vi "PIMAX_2.vi"() -> ()   [LabVIEW 2018]
uses:
  <vilib>/Enthought/Python Integration Toolkit/api/Console Visibility.ctl
  Global Variables.vi
  <vilib>/Enthought/Python Integration Toolkit/Python Integration Toolkit.lvlib
panel:
  in  "Settings":T1(array[cluster])=[{"Camera Setup"=enum."Imaging", "Acuisition type"=enum."Repetitive", "Gate Width"=10000.0, "Gate Start"=200.0, "# Frames"=1, "Center \nWavelength"=790.0, "# Acquisitions"=100, "Exposures per frame"=10}, {"Camera Setup"=enum."Imaging", "Acuisition type"=enum."Sequential", "Gate Width"=300.0, "Gate Start"=200.0, "# Frames"=20, "Center \nWavelength"=790.0, "# Acquisitions"=10, "Exposures per frame"=10}] {"# Acquisitions" min=1; "# Frames" min=1; "Gate Start" min=1.0 format="%#_13g"; "Gate Width" min=0.5 format="%#_13g"}
  out "Index Values":u32[](array[numeric])
  in  "Experiment Name":string="Imaging"
  in  "Logfile?":bool
  in  "File Path":path=path "F:/Data/Raw Data/2018-11-14/UnspecifiedProj/Temp Dependence/PIMAX_2_400C_3"
  in  "stop":bool
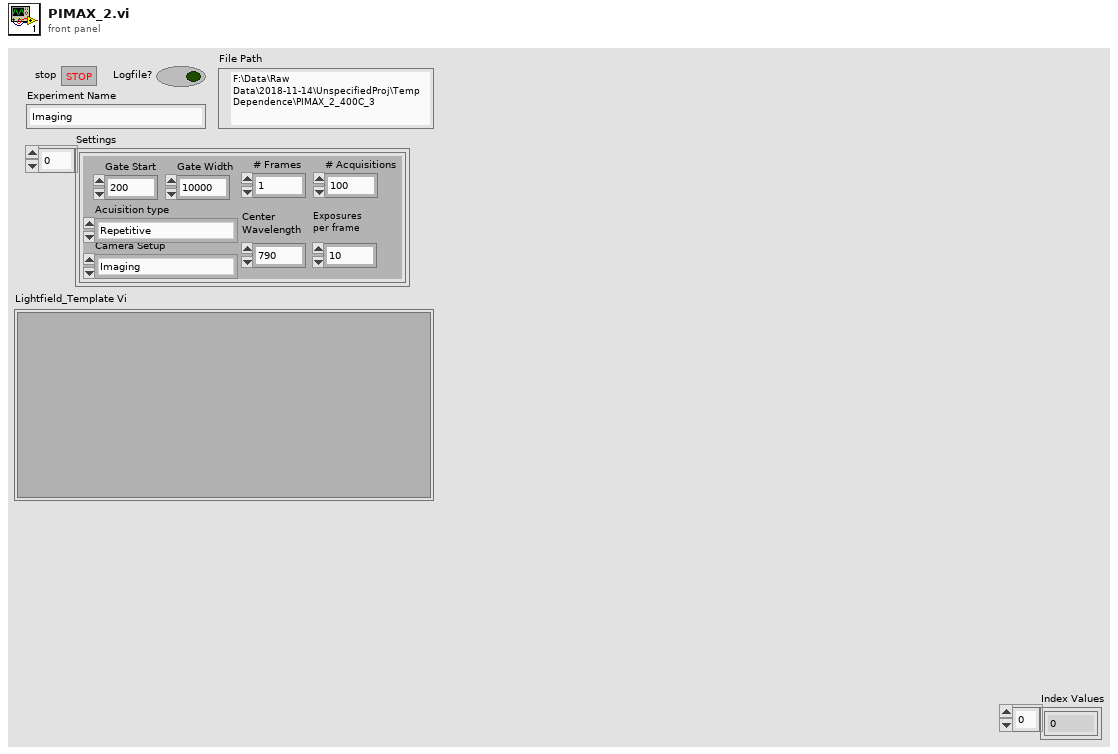
[diagram p1: front panel]
types:
  T1 = cluster{"Camera Setup":enum16{"Imaging", "Spectral"}, "Acuisition type":enum16{"Repetitive", "Sequential"}, "Gate Width":dbl, "Gate Start":dbl, "# Frames":i32, "Center \nWavelength":dbl, "# Acquisitions":i32, "Exposures per frame":i32}[]
  T2 = typedef "Python Integration Toolkit.lvlib/Console Visibility.ctl" = enum16{"Show Console", "Show Console While Running", "Hide Console"}
  T3 = enum32{"Bad", "Idle", "Run top level", "Running"}
  T4 = typedef "Python Integration Toolkit.lvlib/Session ID.ctl" = u64
  T5 = cluster{"Project":u16, "SubFolder":string, "Filename (Meas. Description)":string, "Measurement index":i32}
  T6 = typedef "Python Integration Toolkit.lvlib/Python Objects.ctl" = variant
  T7 = cluster{"Camera Setup":enum16{"Imaging", "Spectral"}, "Acuisition type":enum16{"Repetitive", "Sequential"}, "Gate Width":dbl, "Gate Start":dbl, "# Frames":i32, "Center \nWavelength":dbl, "# Acquisitions":i32, "Exposures per frame":i32}
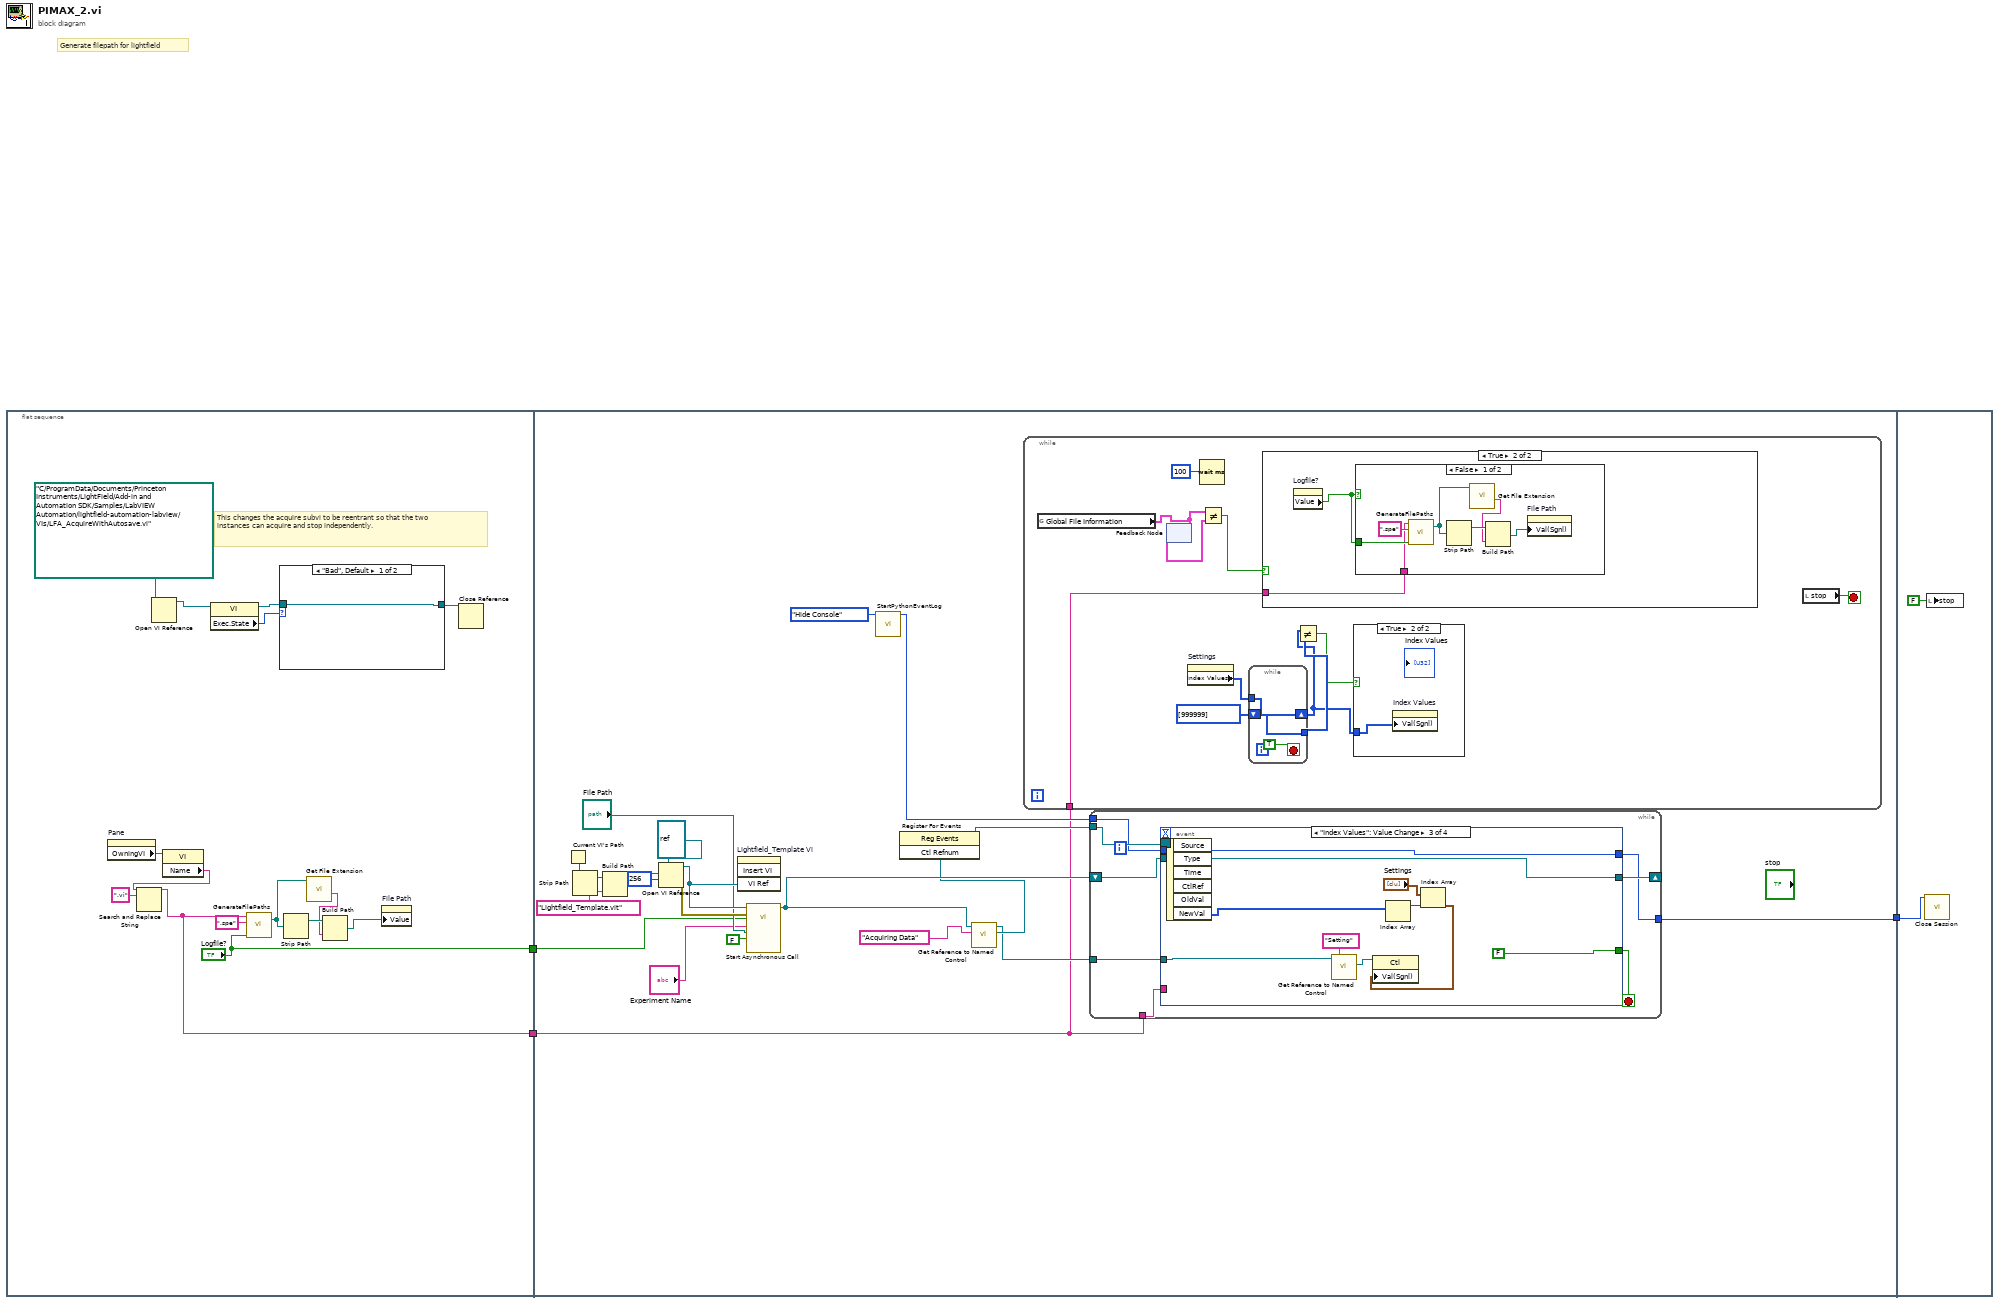
[diagram p0: block diagram]
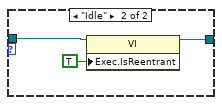
[diagram p2: hidden frame]
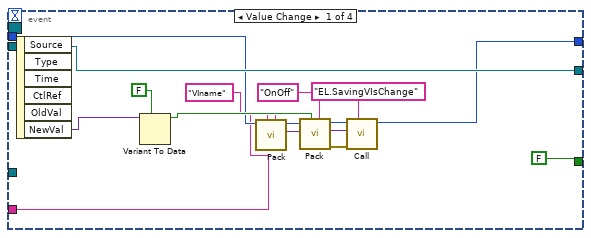
[diagram p6: hidden frame]
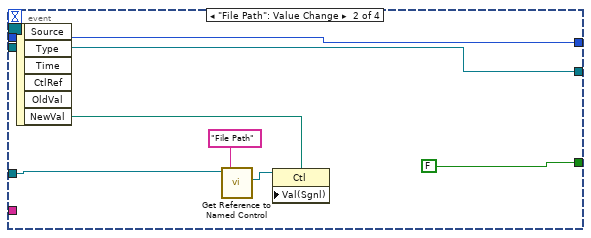
[diagram p7: hidden frame]
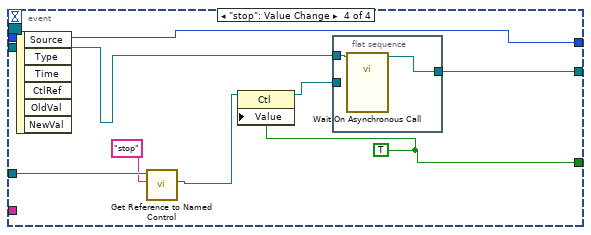
[diagram p8: hidden frame]
diagram:
  # "Generate filepath for lightfield"
  n1 = flat-sequence {
    tunnel: [w5] -> w2
    tunnel: ["Logfile?"] -> w1
    tunnel: [w32] -> w3
    tunnel: w2 -> [w25]
    tunnel: w1 -> [w24]
    tunnel: w3 -> [w119]
    frame #0 {
      # "This changes the acquire subvi to be reentrant so that the two instances can acquire and stop independently."
      n2 = property on="Pane" class="Pane"() -> ("OwningVI"=w8:refnum<vi>)  [unwired: 2 in, 2 out]
      n3 = Open VI Reference(vi path=path "C:/ProgramData/Documents/Princeton Instruments/LightField/Add-in and Automation SDK/Samples/LabVIEW Automation/lightfield-automation-labview/VIs/LFA_AcquireWithAutosave.vi") -> (vi reference=w11:refnum<vi>)  [unwired: 5 in, 1 out]
      n4 = property class="VI"(reference=w8) -> ("Name"=w6:string)  [unwired: 1 in, 2 out]
      n5 = Search and Replace String(input string=w6, search string=".vi") -> (result string=w5:string)  [unwired: 6 in, 3 out]
      n6 = property class="VI"(reference=w11) -> (reference out=w9:refnum<vi>, "Exec.State"=w10:T3)  [unwired: 1 in, 1 out]
      n7 = call "GenerateFilePaths.vi"("Logfile? (F)"="Logfile?", "Extension (.tdms)"=".spe" ("Extension"), "Device Name"=w5) -> ("Path"=w15:path)  [unwired: 2 in]
      n8 = case shown="\"Bad\", Default" w10 {
        tunnel: [w19 w21] -> w17
        tunnel: w9 -> [w19 w20]
        frame "Bad", Default {
        }
        frame "Idle" {
          n9 = property class="VI"(reference=w20, "Exec.IsReentrant"=TRUE ("Execution:Is Reentrant")) -> (reference out=w21:refnum<vi>)  [unwired: 1 in, 1 out]
        }
      }
      n10 = Strip Path(path=w15) -> (stripped path=w14:path)  [unwired: 1 out]
      n11 = call <vilib>:"Get File Extension.vi"("file"=w15) -> ("filename without extension"=w13:string)  [unwired: 6 in, 4 out]
      n12 = Build Path(base path=w14, name or relative path=w13) -> (appended path=w12:path)
      n13 = property on="File Path" class="Path"("Value"=w12) -> ()  [unwired: 2 in, 2 out]
      n14 = Close Reference(reference=w17) -> ()  [unwired: 1 in, 1 out]
    }
    frame #1 {
      n15 = Current VI's Path() -> (path=w42:path)
      n16 = Strip Path(path=w42) -> (stripped path=w43:path)  [unwired: 1 out]
      n17 = Build Path(base path=w43, name or relative path="Lightfield_Template.vit") -> (appended path=w39:path)
      n18 = Open VI Reference(type specifier VI Refnum (for type only)=refnum<vi> refnum, vi path=w39, options=256) -> (vi reference=w38:refnum<vi>, error out=w37:errorcluster)  [unwired: 1 in, 2 out]
      n19 = invoke on="Lightfield_Template Vi" class="SubPnl" method="Insert VI"("VI Ref"=w38) -> ()  [unwired: 3 in, 4 out]
      n20 = call-by-ref "Start Asynchronous Call"(reference=w38, error in=w37, "Add Time to filename"=w24, "Single Run"=FALSE, "File Path"="File Path", "Experiment Name"="Experiment Name") -> (reference out=w31:refnum<vi>)  [unwired: 8 in, 1 out]
      n21 = call "StartPythonEventLog.vi"("Console Visibility"=Console_Visibility."Hide Console") -> ("Session ID out"=w33:T4)  [unwired: 10 in]
      n22 = call "Get Reference to Named Control.vi"("Control Name"="Acquiring Data" ("element"), "Front Panel Ref"=w31) -> ("Ctl Refnum"=w29:refnum<vi>, "Panel Ref Out"=w28:refnum<vi>)  [unwired: 7 in, 1 out]
      n23 = register-events(w29) -> (reference out=w34:refnum<event-registration>)  [unwired: 2 in, 1 out]
      n24 = while {
        tunnel: w25 -> [w49]
        stop <- w54 stop-if-true
        n25 = global read "Global Variables.vi" "Global File Information"() -> (w52:T5)
        n26 = feedback #1() -> (w51:T5)  [unwired: 1 in]
        n27 = feedback-in #1(w52) -> ()
        n28 = property on="Settings" class="Arr (strict)"() -> ("Index Values"=w47:u32[])  [unwired: 2 in, 2 out]
        n29 = Wait (ms)(milliseconds to wait=100) -> ()  [unwired: 1 out]
        n30 = Not Equal?(x=w52, y=w51) -> (x != y?=w50:bool)
        n31 = while {
          tunnel: w47 -> [w58]
          shift-right: [w58] -> w44
          shift-left: u32[] [999999] ("Index Values") -> [w57]
          tunnel: [w57] -> w48
          stop <- TRUE stop-if-true
        }
        n32 = case shown="True" w50 {
          tunnel: w49 -> [_ w59]
          frame False {
          }
          frame True {
            n33 = property on="Logfile?" class="Bool (strict)"() -> ("Value"=w60:bool)  [unwired: 2 in, 2 out]
            n34 = case shown="False" w60 {
              tunnel: w60 -> [w63 _]
              tunnel: w59 -> [w61 _]
              frame False {
                n35 = call "GenerateFilePaths.vi"("Logfile? (F)"=w63, "Extension (.tdms)"=".spe" ("Extension"), "Device Name"=w61) -> ("Path"=w66:path)  [unwired: 2 in]
                n36 = Strip Path(path=w66) -> (stripped path=w65:path)  [unwired: 1 out]
                n37 = call <vilib>:"Get File Extension.vi"("file"=w66) -> ("filename without extension"=w64:string)  [unwired: 6 in, 4 out]
                n38 = Build Path(base path=w65, name or relative path=w64) -> (appended path=w62:path)
                n39 = property on="File Path" class="Path"("Val(Sgnl)"=w62) -> ()  [unwired: 2 in, 2 out]
              }
              frame True {
              }
            }
          }
        }
        n40 = Not Equal?(x=w44, y=w48) -> (x != y?=w46:bool)
        n41 = case shown="True" w46 {
          tunnel: w44 -> [_ w55]
          frame False {
          }
          frame True {
            n42 = property on="Index Values" class="Arr (strict)"("Val(Sgnl)"=w55) -> ()  [unwired: 2 in, 2 out]
          }
        }
        n43 = local read "stop"() -> (w54:bool)
      }
      n44 = while {
        shift-right: [w73] -> _
        shift-left: w31 -> [w74]
        tunnel: w34 -> [w72]
        tunnel: w33 -> [w71]
        tunnel: [w70] -> w32
        tunnel: w28 -> [w69]
        tunnel: w25 -> [w68]
        stop <- w75 stop-if-true
        n45 = event shown="[2] \"Index Values\": Value Change" {
          selector: w72 -> [_ _ _ _]
          dyn-events: _ -> [_ _ _ _]
          timeout: _ -> [_ _ _ _]
          tunnel: [FALSE FALSE FALSE w116] -> w75
          tunnel: w74 -> [w90 w96 w107 w115]
          tunnel: [w90 w96 w107 w114] -> w73
          tunnel: w71 -> [w84 w92 w103 w109]
          tunnel: [w77 w92 w103 w109] -> w70
          tunnel: w69 -> [_ w94 w105 w112]
          tunnel: w68 -> [w76 _ _ _]
          event Value Change {
            n46 = event-data() -> ("NewVal"=w89:variant)  [unwired: 1 in, 5 out]
            n47 = Variant To Data(type=FALSE, Variant=w89) -> (data=w87:bool)  [unwired: 1 in, 1 out]
            n48 = call <vilib>:"Pack.vi"("Keyword Name"="VIname", "Argument"=w76, "Session ID"=w84) -> ("Python Object References Out"=w79:T6, "Session ID out"=w83:T4)  [unwired: 6 in, 1 out]
            n49 = call <vilib>:"Pack.vi"("Keyword Name"="OnOff", "Argument"=w87, "Python Object References In"=w79, "Session ID"=w83) -> ("error out"=w82:errorcluster, "Python Object References Out"=w81:T6, "Session ID out"=w80:T4)  [unwired: 5 in]
            n50 = call <vilib>:"Call.vi"("Function or Method Name"="EL.SavingVIsChange", "error in (no error)"=w82, "Python Object References In"=w81, "Session ID"=w80) -> ("Session ID out"=w77:T4)  [unwired: 5 in, 2 out]
          }
          event "File Path": Value Change {
            n51 = event-data() -> ("NewVal"=w98:path)  [unwired: 1 in, 5 out]
            n52 = call "Get Reference to Named Control.vi"("Control Name"="File Path" ("element"), "Front Panel Ref"=w94) -> ("Ctl Refnum"=w93:refnum<vi>)  [unwired: 7 in, 2 out]
            n53 = property class="Ctl"(reference=w93, "Val(Sgnl)"=w98) -> ()  [unwired: 1 in, 2 out]
          }
          event "Index Values": Value Change {
            n54 = event-data() -> ("NewVal"=w101:u32[])  [unwired: 1 in, 5 out]
            n55 = call "Get Reference to Named Control.vi"("Control Name"="Setting" ("element"), "Front Panel Ref"=w105) -> ("Ctl Refnum"=w104:refnum<vi>)  [unwired: 7 in, 2 out]
            n56 = Index Array(array=w101) -> (element=w102:u32)  [unwired: 1 in]
            n57 = Index Array(array="Settings", index=w102) -> (element=w99:T7)
            n58 = property class="Ctl"(reference=w104, "Val(Sgnl)"=w99) -> ()  [unwired: 1 in, 2 out]
          }
          event "stop": Value Change {
            w116 = TRUE
            n59 = event-data() -> ()  [unwired: 1 in, 6 out]
            n60 = call "Get Reference to Named Control.vi"("Control Name"="stop", "Front Panel Ref"=w112) -> ("Ctl Refnum"=w110:refnum<vi>)  [unwired: 7 in, 2 out]
            n61 = property class="Ctl"(reference=w110, "Value"=w116) -> (reference out=w113:refnum<vi>)  [unwired: 1 in, 1 out]
            n62 = flat-sequence {
              tunnel: w115 -> [w118]
              tunnel: w113 -> [_]
              tunnel: [w117] -> w114
              frame #0 {
                n63 = call-by-ref "Wait On Asynchronous Call"(reference=w118) -> (reference out=w117:refnum<vi>)  [unwired: 13 in, 1 out]
              }
            }
          }
        }
      }
    }
    frame #2 {
      n64 = call <vilib>:"Close Session.vi"("Session ID"=w119) -> ()  [unwired: 10 in, 1 out]
      n65 = local write "stop"(FALSE ("stop")) -> ()
    }
  }
